vi "Save Confluence Printer Settings.vi"(8 "Error in":errorcluster caption="Error in (no error)", 10 "Confluence Printer Settings":T1={"Expand Structures"={"VI Member"={"By Folder Expand"=TRUE, "By Tree Expand"=TRUE, "By List Expand"=TRUE, "Methods Expand"=TRUE, "Controls Expand"=TRUE}, "Control Member"={"By Folder Expand"=TRUE, "By Tree Expand"=TRUE, "By List Expand"=TRUE, "Controls Expand"=TRUE}, "Interface"={"List Expand"=TRUE, "Controls Expand"=TRUE, "Methods Expand"=TRUE, "Inheritance Expand"=TRUE}, "Library"={"By Folder Expand"=TRUE, "By Tree Expand"=TRUE, "By List Expand"=TRUE, "Controls Expand"=TRUE, "Methods Expand"=TRUE, "Inheritance Expand"=TRUE}, "Class"={"By Folder Expand"=TRUE, "By Tree Expand"=TRUE, "By List Expand"=TRUE, "CPD Expand"=TRUE, "Controls Expand"=TRUE, "Methods Expand"=TRUE, "Set Accessors Expand"=TRUE, "Get Accessors Expand"=TRUE, "Inheritance Expand"=TRUE}}, "Sortable Tables"=TRUE, "Table Column Ordering"={"Class List"={"Minimal"=[], "Standard"=[], "Full"=[]}, "Library List"={"Minimal"=[], "Standard"=[], "Full"=[]}, "Control FP"={"Minimal"=[], "Standard"=[], "Full"=[]}, "Library Control Files"={"Minimal"=[], "Standard"=[], "Full"=[]}, "UI Methods"={"Minimal"=[], "Standard"=[], "Full"=[]}, "Method List"={"Minimal"=[], "Standard"=[], "Full"=[]}, "Interface Methods"={"Minimal"=[], "Standard"=[], "Full"=[]}, "LLB Methods"={"Minimal"=[], "Standard"=[], "Full"=[]}, "Library Methods"={"Minimal"=[], "Standard"=[], "Full"=[]}, "Class Methods"={"Minimal"=[], "Standard"=[], "Full"=[]}}} caption="Doc Options", 11 "Settings Path":path) -> (0 "Error out":errorcluster)   [LabVIEW 2023, in "VIDoc Printer - Confluence.lvlib" / "VIDoc Settings - Confluence.lvclass"]
uses:
  VIDoc Settings - Confluence.lvclass
  e450ed71-4968-4477-8672-58ac8a0708d9.vi
  VIDoc Settings/VIDoc Settings.lvclass
  Confluence Printer Settings Cluster.ctl
  Class Info Column.ctl
  Control Info Column.ctl
  VI Info Column.ctl
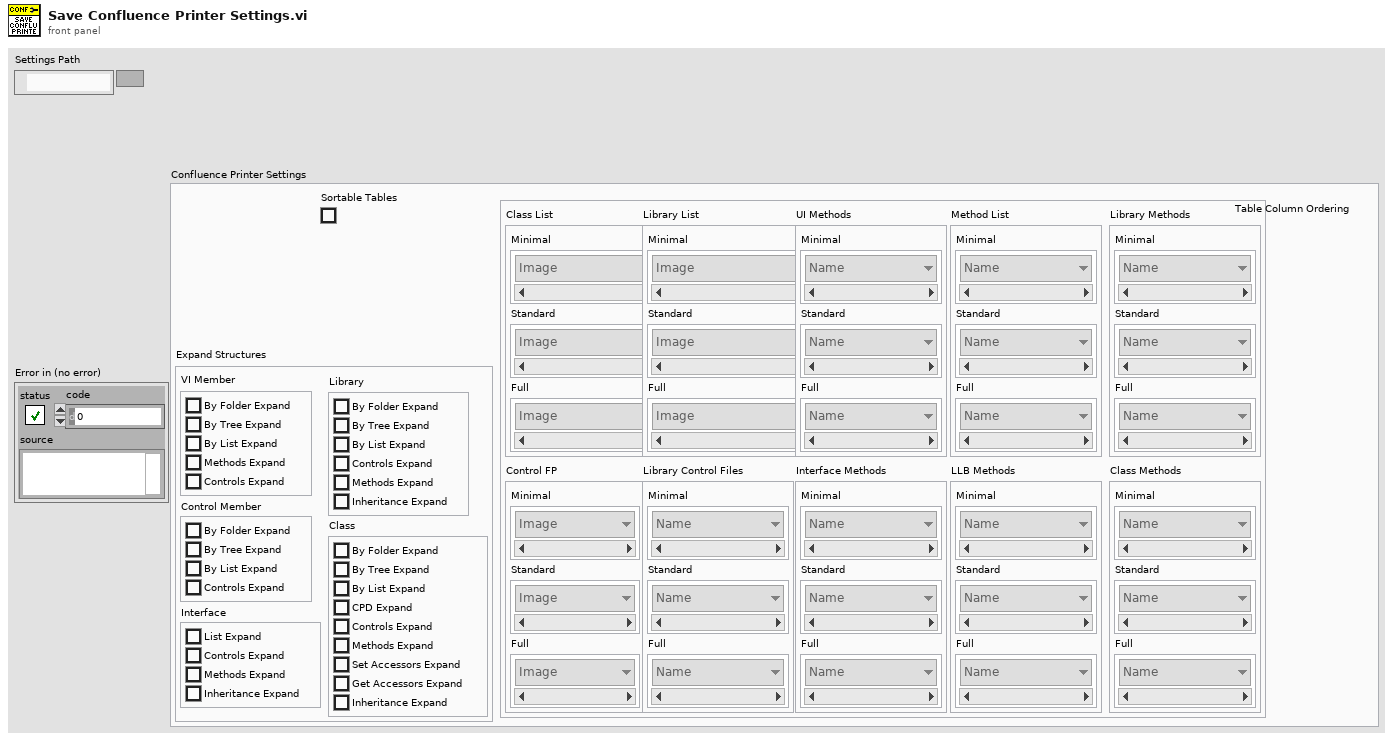
[diagram p1: front panel]
types:
  T1 = typedef "VIDoc Printer - Confluence.lvlib/VIDoc Settings - Confluence.lvclass/Confluence Printer Settings Cluster.ctl" = cluster{"Expand Structures":cluster{"VI Member":cluster{"By Folder Expand":bool, "By Tree Expand":bool, "By List Expand":bool, "Methods Expand":bool, "Controls Expand":bool}, "Control Member":cluster{"By Folder Expand":bool, "By Tree Expand":bool, "By List Expand":bool, "Controls Expand":bool}, "Interface":cluster{"List Expand":bool, "Controls Expand":bool, "Methods Expand":bool, "Inheritance Expand":bool}, "Library":cluster{"By Folder Expand":bool, "By Tree Expand":bool, "By List Expand":bool, "Controls Expand":bool, "Methods Expand":bool, "Inheritance Expand":bool}, "Class":cluster{"By Folder Expand":bool, "By Tree Expand":bool, "By List Expand":bool, "CPD Expand":bool, "Controls Expand":bool, "Methods Expand":bool, "Set Accessors Expand":bool, "Get Accessors Expand":bool, "Inheritance Expand":bool}}, "Sortable Tables":bool, "Table Column Ordering":cluster{"Class List":cluster{"Minimal":T2[], "Standard":T2[], "Full":T2[]}, "Library List":cluster{"Minimal":T2[], "Standard":T2[], "Full":T2[]}, "Control FP":cluster{"Minimal":T3[], "Standard":T3[], "Full":T3[]}, "Library Control Files":cluster{"Minimal":T4[], "Standard":T4[], "Full":T4[]}, "UI Methods":cluster{"Minimal":T4[], "Standard":T4[], "Full":T4[]}, "Method List":cluster{"Minimal":T4[], "Standard":T4[], "Full":T4[]}, "Interface Methods":cluster{"Minimal":T4[], "Standard":T4[], "Full":T4[]}, "LLB Methods":cluster{"Minimal":T4[], "Standard":T4[], "Full":T4[]}, "Library Methods":cluster{"Minimal":T4[], "Standard":T4[], "Full":T4[]}, "Class Methods":cluster{"Minimal":T4[], "Standard":T4[], "Full":T4[]}}}
  T2 = typedef "VIDoc Printer - Confluence.lvlib/VIDoc Settings - Confluence.lvclass/Class Info Column.ctl" = enum16{"Image", "Name", "Description", "Version", "Last Change", "Author", "Commit Hash", "Branch", "Qualified Name", "TransferMustOverrides", "ChildRefsRestricted"}
  T3 = typedef "VIDoc Printer - Confluence.lvlib/VIDoc Settings - Confluence.lvclass/Control Info Column.ctl" = enum16{"Image", "Name", "Description", "Caption", "Tip Strip", "Data Type", "Key Toggle"}
  T4 = typedef "VIDoc Printer - Confluence.lvlib/VIDoc Settings - Confluence.lvclass/VI Info Column.ctl" = enum16{"Name", "Conpane", "BD", "FP", "VI Icon", "Description", "Reentrant", "Inline", "Auto Error", "Compiled", "Code Complexity", "Data Size", "Debug", "Priority", "Rev", "Minimum Size", "Title", "FP Behavior", "FP Closeable", "Author", "Commit Hash", "Last Change", "Branch", "Scope", "Type", "Dispatch", "Must Override", "Must Use Parent", "Structure Tree"}
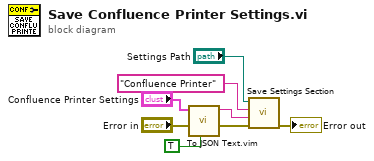
[diagram p0: block diagram]
diagram:
  n1 = call "To JSON Text.vim"("Pretty Print?"=TRUE, "error in (no error)"="Error in", "Anything"="Confluence Printer Settings") -> ("error out"=w6:errorcluster, "<JSON>"=w4:string)  [unwired: 7 in]
  n2 = call "Save Settings Section.vi"("Error in"=w6, "JSON Object"=w4, "Section Name"="Confluence Printer", "JSON Settings Path"="Settings Path") -> ("Error out"=→"Error out":errorcluster)  [unwired: 7 in]
